vi "Initialize and Run Finite VI.vi"(8 "error in (no error)":errorcluster, 10 "Settings":T1(array[cluster]), 11 "Initialization VI":path) -> (0 "error out":errorcluster, 3 "VI out":refnum<vi>)   [LabVIEW 2019, in "Simple SysDef API.lvlib"]
uses:
  <userlib>/SimpleSysDef/Simple SysDef API.lvlib
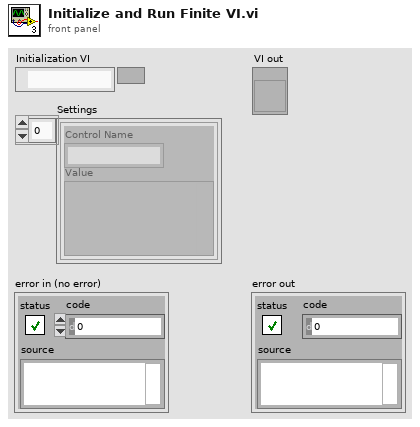
[diagram p1: front panel]
types:
  T1 = cluster{"Control Name":string, "Value":variant}[]
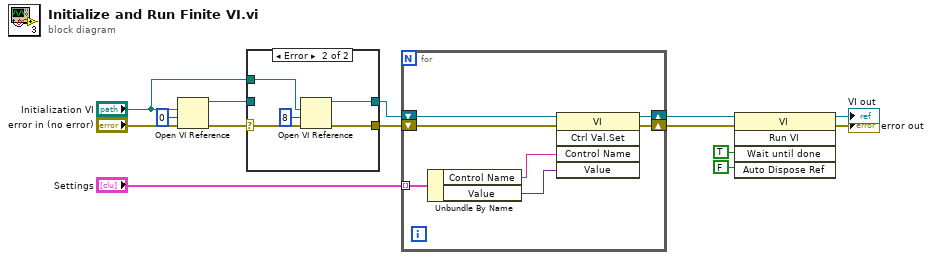
[diagram p0: block diagram]
diagram:
  n1 = Open VI Reference(vi path="Initialization VI", options=0, error in (no error)="error in (no error)") -> (vi reference=w3:refnum<vi>, error out=w2:errorcluster)  [unwired: 3 in]
  n2 = case shown="Error" w2 {
    selector: w2 -> [w15 w20]
    tunnel: w3 -> [w16 _]
    tunnel: [w16 w18] -> w9
    tunnel: [w15 w19] -> w10
    tunnel: "Initialization VI" -> [_ w17]
    frame No Error {
    }
    frame Error {
      n3 = Open VI Reference(vi path=w17, options=8, error in (no error)=w20) -> (vi reference=w18:refnum<vi>, error out=w19:errorcluster)  [unwired: 3 in]
    }
  }
  n4 = for {
    shift-right: [w25] -> w12
    shift-left: w9 -> [w28]
    shift-right: [w26] -> w11
    shift-left: w10 -> [w27]
    tunnel: "Settings" -> [w24] mode=indexing
    n5 = Unbundle By Name(w24) -> ("Control Name"=w23:string, "Value"=w22:variant)
    n6 = invoke class="VI" method="Ctrl Val.Set"(reference=w28, error in=w27, "Control Name"=w23, "Value"=w22) -> (reference out=w25:refnum<vi>, error out=w26:errorcluster)  [unwired: 1 in, 3 out]
  }
  n7 = invoke class="VI" method="Run VI"(reference=w12, error in=w11, "Wait until done"=TRUE ("Wait Until Done"), "Auto Dispose Ref"=FALSE ("Auto Dispose Reference")) -> (reference out=→"VI out":refnum<vi>, error out=→"error out":errorcluster)  [unwired: 1 in, 3 out]
